vi "NI_FPGA_PPG.load with description.vi"(0 "i ref in":refnum<vi>, 1 "cmd_data_string":string, 2 "cmd_data_description_string":string, 3 "ms timeout (10000)":i32=10000, 4 "channel_description_string":string, 5 "error in (no error)":errorcluster) -> (14 "i ref out":refnum<vi>, 17 "timed out":bool, 19 "error out":errorcluster)   [LabVIEW 2014, in "NI_FPGA_PPG.lvlib"]
doc: "Loads complete command sequence (see command syntax) inlcuding descriptions to the FPGA target.\n\nLicense Agreement for this software:\n\nCopyright (C) 2009\nFalk Ziegler\nInstitut für Physik\nErnst-Moritz-Arndt Universität\nFelix-Hausdorff-Str. 6\n17487 Greifswald\n\nContact: Falk Ziegler, ziegler@physik.uni-greifswald.de\n\nThis program is free software: you can redistribute it and/or modify it under the terms of the GNU General Public License as published by the Free Software Foundation, either version 3 of the License, or (at your option) any later version.\n\nThis program is distributed in the hope that it will be useful, but WITHOUT ANY WARRANTY; without even the implied warranty of MERCHANTABILITY or FITNESS FOR A PARTICULAR PURPOSE. See the GNU General Public License for more details.\n\nYou should have received a copy of the GNU General Public License along with this program. If not, see <http://www.gnu.org/licenses/>.\n\nFor all questions and ideas contact: ziegler@physik.uni-greifswald.de or d.beck@gsi.de\nLast update: 01-Sep-2009"
uses:
  NI_FPGA_PPG.lvlib
  CSCore/CSApplicationBaseClasses/DeviceBase/DeviceBase.lvlib
  CSinstr.lib/NI_FPGA_PPG/host/instrumentDriver/NI-FPGA_PPG_Driver.lvlib
  CSCore/CSSystem/CoreLib/CoreLib.lvlib
  CSlibraries/UtilityLib/UtilityLib.lvlib
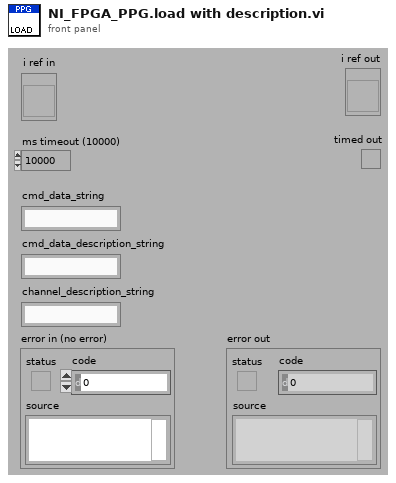
[diagram p1: front panel]
types:
  T1 = typedef "NI_FPGA_PPG.lvlib/NI_FPGA_PPG.i attribute.ctl" = cluster{"dim_service_id":cluster{"dim_actual_device_status":i32, "dim_event_data":i32, "dim_cmd_data":i32, "dim_cmd_data _description":i32, "dim_channel_description":i32}, "VISA":refnum<visa-resource-name>, "actual_device_status":i32, "event_data_id":i32, "pdc_enabled":bool, "pdc_timestamp":u32, "cmd_data_string":string, "cmd_data_size":i32, "cmd_data_description_string":string, "cmd_data_description_size":i32, "channel_description_string":string, "channel_description_size":i32}
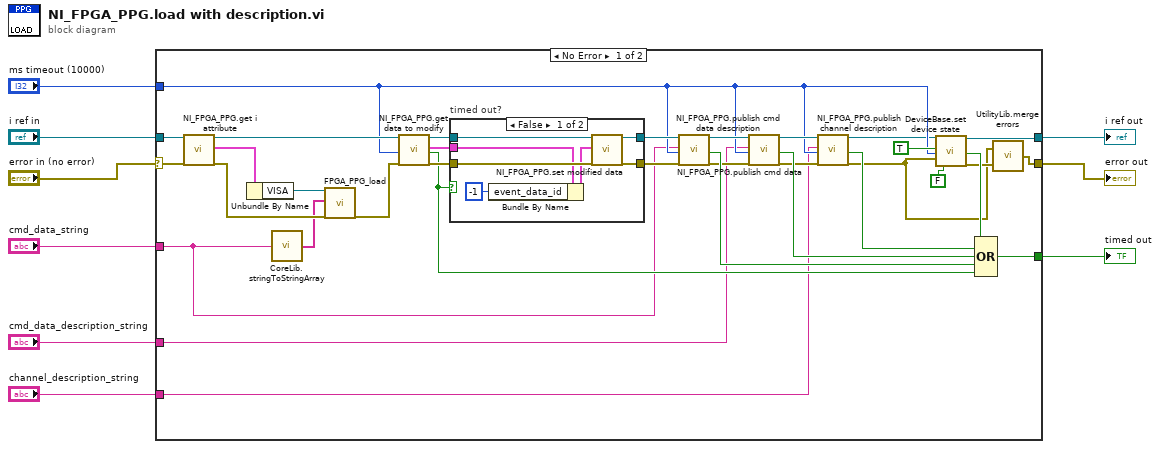
[diagram p0: block diagram]
diagram:
  n1 = case shown="No Error" "error in (no error)" {
    selector: "error in (no error)" -> [w42 w53]
    tunnel: "i ref in" -> [w43 w54]
    tunnel: [w36 w54] -> w7
    tunnel: [w10 w53] -> w6
    tunnel: "ms timeout (10000)" -> [w20 _]
    tunnel: "cmd_data_string" -> [w15 _]
    tunnel: [w29 _] -> w3
    tunnel: "cmd_data_description_string" -> [w14 _]
    tunnel: "channel_description_string" -> [w13 _]
    frame No Error {
      n2 = call "NI_FPGA_PPG.get i attribute.vi"("i ref in"=w43, "error in (no error)"=w42) -> ("i ref out"=w35:refnum<vi>, "i attribute"=w41:T1, "error out"=w39:errorcluster)  [unwired: 15 in]
      n3 = Unbundle By Name(w41) -> ("VISA"=w40:refnum<visa-resource-name>)
      n4 = call "CoreLib.stringToStringArray.vi"("String"=w15) -> ("Array"=w17:string[])
      n5 = call "FPGA_PPG_load.vi"("resource_in"=w40, "command_lines"=w17, "error in (no error)"=w39) -> ("error out"=w16:errorcluster)  [unwired: 15 in, 1 out]
      n6 = call "NI_FPGA_PPG.get data to modify.vi"("i ref in"=w35, "ms timeout (10000)"=w20, "error in (no error)"=w16) -> ("i ref out"=w34:refnum<vi>, "i attribute"=w32:T1, "timed out"=w30:bool, "error out"=w33:errorcluster)  [unwired: 13 in]
      n7 = case "timed out?" shown="False" w30 {
        tunnel: w34 -> [w50 w52]
        tunnel: w33 -> [w49 w51]
        tunnel: w32 -> [w48 _]
        tunnel: [w45 w52] -> w28
        tunnel: [w44 w51] -> w27
        frame False {
          n8 = Bundle By Name(cluster=w48, "event_data_id"=-1) -> (w47:T1)
          n9 = call "NI_FPGA_PPG.set modified data.vi"("i ref in"=w50, "i attribute"=w47, "error in (no error)"=w49) -> ("i ref out"=w45:refnum<vi>, "error out"=w44:errorcluster)  [unwired: 15 in]
        }
        frame True {
        }
      }
      n10 = call "NI_FPGA_PPG.publish cmd data.vi"("i ref in"=w28, "cmd_data_string"=w15, "ms timeout (10000)"=w20, "error in (no error)"=w27) -> ("i ref out"=w24:refnum<vi>, "timed out"=w26:bool, "error out"=w25:errorcluster)  [unwired: 13 in]
      n11 = call "NI_FPGA_PPG.publish cmd data description.vi"("i ref in"=w24, "cmd_data_string"=w14, "ms timeout (10000)"=w20, "error in (no error)"=w25) -> ("i ref out"=w22:refnum<vi>, "timed out"=w23:bool, "error out"=w21:errorcluster)  [unwired: 13 in]
      n12 = call "NI_FPGA_PPG.publish channel description.vi"("i ref in"=w22, "channel_description"=w13, "ms timeout (10000)"=w20, "error in (no error)"=w21) -> ("i ref out"=w19:refnum<vi>, "timed out"=w18:bool, "error out"=w11:errorcluster)  [unwired: 13 in]
      n13 = call "DeviceBase.set device state.vi"("i ref in"=w19, "implicit"=TRUE, "ms timeout (10000)"=w20, "device error"=w11, "mayResetError (FALSE)"=FALSE) -> ("i ref out"=w36:refnum<vi>, "timed out"=w31:bool, "error out"=w12:errorcluster)  [unwired: 12 in]
      n14 = Compound Arithmetic op=OR(w31, w18, w23, w26, w30) -> (w29:bool)
      n15 = call "UtilityLib.merge errors.vi"("error2 (no error)"=w12, "error1 (no error)"=w11) -> ("error out"=w10:errorcluster)
    }
    frame Error {
    }
  }
  "error out" <- w6
  "i ref out" <- w7
  "timed out" <- w3
